vi "Get IMAQ Ctrl Ref Index.vi"(0 "Image Idx":i32, 11 "Error In":errorcluster) -> (4 "Generic Ref":refnum<vi>, 15 "Error Out":errorcluster)   [LabVIEW 2020]
uses:
  <vilib>/vision/Image Controls.llb/IMAQ Image.ctl
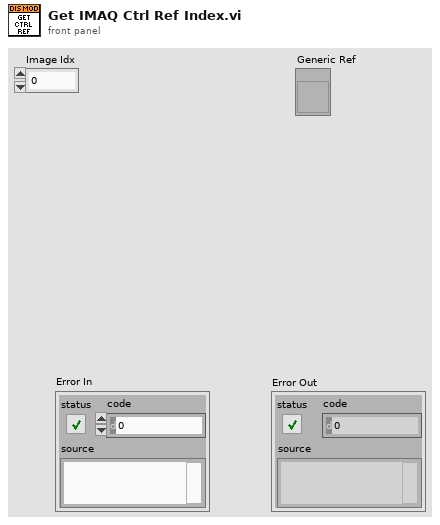
[diagram p1: front panel]
types:
  T1 = typedef "IMAQ Image.ctl" = refnum<image>
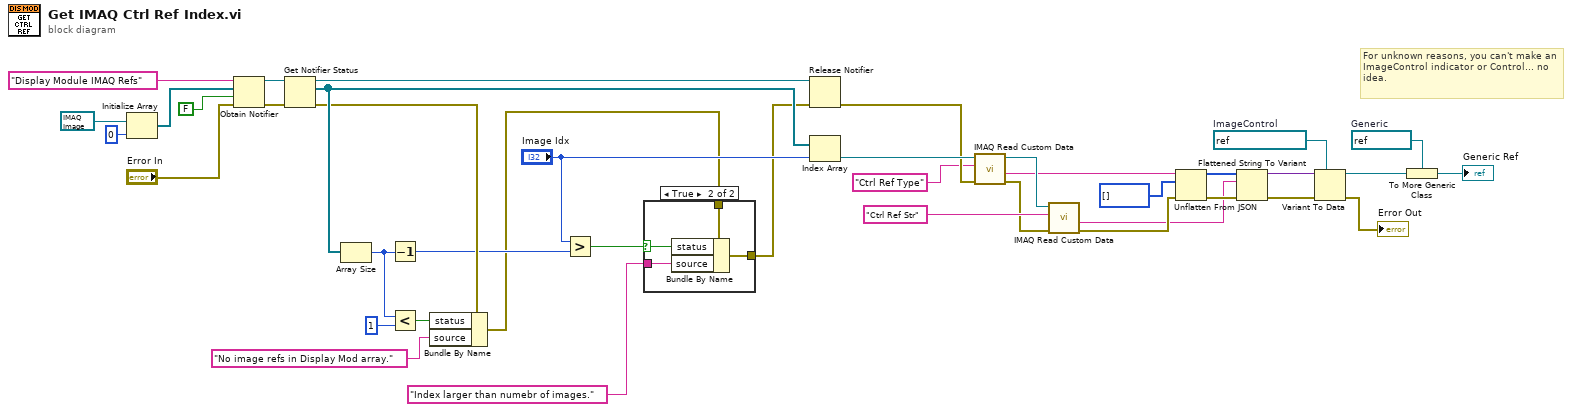
[diagram p0: block diagram]
diagram:
  w2 = refnum<vi> refnum  # Generic
  w6 = refnum<vi> refnum  # ImageControl
  # "For unknown reasons, you can't make an ImageControl indicator or Control... no idea."
  n1 = Initialize Array(T1 refnum ("New Image"), 0 ("dimension size")) -> (w36:T1[])
  n2 = Obtain Notifier(name (unnamed)="Display Module IMAQ Refs", notification data type=w36, create if not found? (T)=FALSE, error in (no error)="Error In") -> (notifier out=w35:refnum<notifier>, error out=w34:errorcluster)  [unwired: 1 out]
  n3 = Get Notifier Status(notifier=w35, error in (no error)=w34) -> (notifier out=w33:refnum<notifier>, current notification=w29:T1[], error out=w28:errorcluster)  [unwired: 2 out]
  n4 = Array Size(array=w29) -> (size(s)=w24:i32)
  n5 = Decrement(x=w24) -> (x-1=w23:i32)
  n6 = Less?(x=w24, y=1) -> (x < y?=w26:bool)
  n7 = Bundle By Name(cluster=w28, "status"=w26, "source"="No image refs in Display Mod array.") -> (w21:errorcluster)
  n8 = Greater?(x="Image Idx", y=w23) -> (0:w19:bool)
  n9 = case shown="True" w19 {
    selector: w19 -> [_ w43]
    tunnel: w21 -> [w41 w45]
    tunnel: "Index larger than numebr of images." ("source") -> [_ w44]
    tunnel: [w41 w42] -> w18
    frame False {
    }
    frame True {
      n10 = Bundle By Name(cluster=w45, "status"=w43, "source"=w44) -> (w42:errorcluster)
    }
  }
  n11 = Release Notifier(notifier=w33, error in (no error)=w18) -> (error out=w30:errorcluster)  [unwired: 1 in, 2 out]
  n12 = Index Array(array=w29, index="Image Idx") -> (element=w31:T1)
  n13 = call "IMAQ Read Custom Data"("error in (no error)"=w30, "Key"="Ctrl Ref Type", "Image"=w31) -> ("error out"=w14:errorcluster, "Custom Data Out"=w13:string, "Image (duplicate)"=w16:T1)  [unwired: 6 in]
  n14 = call "IMAQ Read Custom Data"("error in (no error)"=w14, "Key"="Ctrl Ref Str", "Image"=w16) -> ("error out"=w11:errorcluster, "Custom Data Out"=w8:string)  [unwired: 6 in, 1 out]
  n15 = Unflatten From JSON(JSON string=w13, type and defaults=i16[] [], error in (no error)=w11) -> (value=w10:i16[], error out=w9:errorcluster)  [unwired: 4 in]
  n16 = Flattened String To Variant(4:w9, 6:w8, 7:w10) -> (0:w5:errorcluster, 3:w7:variant)
  n17 = Variant To Data(error in=w5, type=w6, Variant=w7) -> (data=w3:refnum<vi>, error out=→"Error Out":errorcluster)
  n18 = To More Generic Class(target class=w2, reference=w3) -> (generic class reference=→"Generic Ref":refnum<vi>)
